vi "Set gate mode.vi"(8 "error in (no error)":errorcluster, 9 "Mode (def: CW)":T1, 10 "Gate (def: A)":T2, 11 "VISA resource name":refnum<visa-resource-name>) -> (0 "error out":errorcluster, 3 "VISA resource name out":refnum<visa-resource-name>)   [LabVIEW 2009, in "SR400.lvlib"]
doc: "GM i { ,j }\nThe GM command sets and reads the gate modes. i\n= 0 or 1 designates A gate or B gate and is\nrequired. If j is included, the selected gate is set to\nCW, j=0, or FIXED, j=1, or SCAN, j=2. If j is\nabsent, the mode of gate i is returned. The mode\nmay be changed during a scan. If it is changed to\nSCAN, the delay begins scanning from the start\nposition on the next count period. If it is changed\nto FIXED, the delay returns to the start position\nimmediately. If it is changed to CW, the gate\nimmediately changes to continuously on."
uses:
  SR400.lvlib
  Typedefs.llb/Gate.ctl
  Typedefs.llb/Gate Mode.ctl
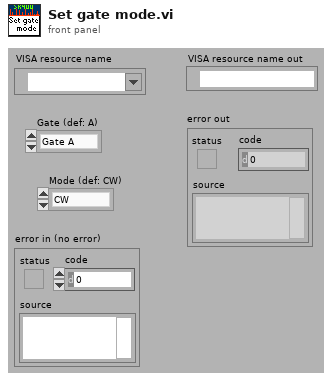
[diagram p1: front panel]
types:
  T1 = typedef "SR400.lvlib/Gate Mode.ctl" = enum16{"CW", "Fixed", "Scan"}
  T2 = typedef "SR400.lvlib/Gate.ctl" = enum16{"Gate A", "Gate B"}
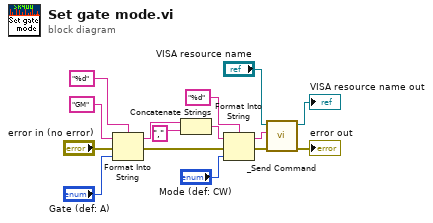
[diagram p0: block diagram]
diagram:
  n1 = Format Into String(format string="%d", initial string="GM" ("command"), error in="error in (no error)", "Gate (def: A)") -> (resulting string=w12:string, error out=w13:errorcluster)
  n2 = Concatenate Strings(w12, "," ("command")) -> (w7:string)
  n3 = Format Into String(format string="%d", initial string=w7, error in=w13, "Mode (def: CW)") -> (resulting string=w4:string, error out=w3:errorcluster)
  n4 = call "_Send Command.vi"("error in (no error)"=w3, "Command"=w4, "VISA resource name"="VISA resource name") -> ("error out"=→"error out":errorcluster, "VISA resource name out"=→"VISA resource name out":refnum<visa-resource-name>)  [unwired: 1 in, 6 out]
